vi "HFRR ADV v06.vi"() -> ()   [LabVIEW 2025] (continued)
            n1283 = local read "TEMP"() -> (w1608:dbl)
            n1284 = local write "FF 3"(w1604) -> ()
            n1285 = Compound Arithmetic op=OR("FRICVALZ 4", "FRICVALZ 3", "FRICVALZ 2") -> (w1601:bool)
            n1286 = case shown="True" w1601 {
              tunnel: w1594 -> [_ w1615]
              frame False {
              }
              frame True {
                w1614 = FALSE ("FRICVALZ")
                n1287 = local write "FRICVALZ 3"(w1614) -> ()
                n1288 = local write "FRICVALZ 2"(w1614) -> ()
                n1289 = local write "FRICVALZ 4"(w1614) -> ()
                "FRICVALZ" <- w1615
              }
            }
            n1290 = Not A Number/Path/Refnum?(number/path/refnum=w1608) -> (NaN/Path/Refnum?=w1607:bool)
            n1291 = Not A Number/Path/Refnum?(number/path/refnum=w1604) -> (NaN/Path/Refnum?=w1606:bool)
            n1292 = Divide(x=w1604, y=1.96) -> (x/y=w1591:dbl)
            n1293 = Compound Arithmetic op=OR(w1607, w1606) -> (w1605:bool)
            n1294 = Not A Number/Path/Refnum?(number/path/refnum=w1591) -> (NaN/Path/Refnum?=w1602:bool)
            n1295 = case shown="True" w1605 {
              frame False {
              }
              frame True {
                n1296 = local write "TEMP"(0.0 ("TEMP")) -> ()
                n1297 = local write "FF 2"(0.0 ("FF 2")) -> ()
                n1298 = local write "reinit"(TRUE ("reinit")) -> ()
              }
            }
            n1299 = Select(t=0.0, s=w1602, f=w1591) -> (s? t:f=w1590:dbl)
            "COF 2" <- w1590
            n1300 = local write "COF 3"(w1590) -> ()
          }
        }
      }
    }
    n1301 = Wait (ms)(milliseconds to wait=u32 50) -> ()  [unwired: 1 out]
    n1302 = local read "Quit"() -> (w1530:bool)
    "Rate" <- 2500.0 ("No of Samples")
  }
  n1303 = while {
    tunnel: w57 -> [_]
    tunnel: [w1642] -> _
    tunnel: [w1618] -> w56
    i -> [w1642]
    stop <- w1618 stop-if-true
    # "C:\\LAB-IQ-NXT\\Scar View.exe"
    n1304 = local read "OK Button 16"() -> (w1631:bool)
    n1305 = local read "Main Tab"() -> (w1624:T2)
    n1306 = local read "service 3"() -> (w1625:bool)
    n1307 = local read "OPEN 6"() -> (w1627:bool)
    n1308 = local read "EDIT 2"() -> (w1629:bool)
    n1309 = flat-sequence {
      frame #0 {
        n1310 = local read "SAVE 2"() -> (w2244:bool)
        n1311 = stacked-sequence {
          frame #0 {
            n1312 = local read "EDIT"() -> (w2298:bool)
            n1313 = case shown="True" w2298 {
              tunnel: [u8 2 ("Disabled") u8 0 ("Disabled")] -> _
              frame False {
                w2300 = FALSE
                n1314 = local write "Password"("") -> ()
                n1315 = property on="SrvM CP" class="Bool (strict)"("Visible"=w2300) -> ()  [unwired: 2 in, 2 out]
                n1316 = property on="message" class="Str"("Visible"=w2300) -> ()  [unwired: 2 in, 2 out]
                n1317 = local write "x = y?"(w2300) -> ()
                n1318 = property on="Password" class="Str"("Visible"=w2300) -> ()  [unwired: 2 in, 2 out]
                n1319 = property on="ENTER THE NEW PASSWORD" class="Str"("Visible"=w2300) -> ()  [unwired: 2 in, 2 out]
                n1320 = property on="ENTER CURRENT PASSWORD" class="Str"("Visible"=w2300) -> ()  [unwired: 2 in, 2 out]
                n1321 = local write "SrvM CP"(w2300) -> ()
              }
              frame True {
                w2303 = TRUE
                n1322 = property on="SrvM CP" class="Bool (strict)"("Visible"=w2303) -> ()  [unwired: 2 in, 2 out]
                n1323 = property on="Password" class="Str"("Visible"=w2303) -> ()  [unwired: 2 in, 2 out]
              }
            }
            "dipl pwd" <- "@143$\n" ("dipl pwd")
          }
          frame #1 {
            # "Gain password"
            n1324 = String To Byte Array(string="ENTER CURRENT PASSWORD") -> (unsigned byte array=w2308:u8[])
            n1325 = Search 1D Array(1D array=w2308, element=u8 10) -> (index of element=w2311:i32)  [unwired: 1 in]
            n1326 = Index Array(array=w2308, index=w2311) -> (element=w2307:u8)
            n1327 = Equal?(x=w2307, y=10) -> (x = y?=w2305:bool)
            n1328 = case shown="True" w2305 {
              frame False {
                n1329 = property on="ENTER THE NEW PASSWORD" class="Str"("Visible"=FALSE) -> ()  [unwired: 2 in, 2 out]
              }
              frame True {
                # "password"
                # "change password logic"
                n1330 = local read "ENTER CURRENT PASSWORD"() -> (w2324:string)
                n1331 = local read "dipl pwd"() -> (w2318:string)
                n1332 = String To Byte Array(string=w2324) -> (unsigned byte array=w2326:u8[])
                n1333 = String To Byte Array(string=w2318) -> (unsigned byte array=w2319:u8[])
                n1334 = Array Size(array=w2326) -> (size(s)=w2323:i32)
                n1335 = Array Size(array=w2319) -> (size(s)=w2321:i32)
                n1336 = for {
                  N: w2323 -> [_]
                  tunnel: w2326 -> [w2350]
                  tunnel: [w2348] -> w2327 mode=indexing
                  tunnel: w2323 -> [w2342]
                  i -> [w2343]
                  n1337 = Decrement(x=w2342) -> (x-1=w2340:i32)
                  n1338 = Equal?(x=w2343, y=w2340) -> (x = y?=w2341:bool)
                  n1339 = Index Array(array=w2350, index=w2343) -> (element=w2344:u8)
                  n1340 = Number To Decimal String(number=w2344) -> (decimal integer string=w2349:string)  [unwired: 1 in]
                  n1341 = Select(t="", s=w2341, f="\r") -> (s? t:f=w2346:string)
                  n1342 = Concatenate Strings(w2349, w2346) -> (w2348:string)
                }
                n1343 = for {
                  N: w2321 -> [_]
                  tunnel: w2319 -> [w2338]
                  tunnel: [w2336] -> w2320 mode=indexing
                  tunnel: w2321 -> [w2333]
                  i -> [w2334]
                  n1344 = Decrement(x=w2333) -> (x-1=w2332:i32)
                  n1345 = Equal?(x=w2334, y=w2332) -> (x = y?=w2331:bool)
                  n1346 = Index Array(array=w2338, index=w2334) -> (element=w2337:u8)
                  n1347 = Number To Decimal String(number=w2337) -> (decimal integer string=w2335:string)  [unwired: 1 in]
                  n1348 = Select(t="", s=w2331, f="\r") -> (s? t:f=w2328:string)
                  n1349 = Concatenate Strings(w2335, w2328) -> (w2336:string)
                }
                n1350 = local read "string"() -> (w2325:string)
                n1351 = Concatenate Strings(w2320) -> (w2314:string)
                n1352 = Concatenate Strings(w2325) -> (w2322:string)
                n1353 = Concatenate Strings(w2327) -> (w2315:string)
                n1354 = Equal?(x=w2315, y=w2322) -> (x = y?=w2317:bool)
                n1355 = Equal?(x=w2315, y=w2314) -> (x = y?=w2313:bool)
                n1356 = Or(x=w2317, y=w2313) -> (x .or. y?=w2316:bool)
                n1357 = case shown="True" w2316 {
                  frame False {
                  }
                  frame True {
                    n1358 = property on="ENTER THE NEW PASSWORD" class="Str"("Visible"=TRUE) -> ()  [unwired: 2 in, 2 out]
                  }
                }
              }
            }
          }
          frame #2 {
            n1359 = String To Byte Array(string="ENTER THE NEW PASSWORD") -> (unsigned byte array=w2353:u8[])
            n1360 = Search 1D Array(1D array=w2353, element=u8 10) -> (index of element=w2357:i32)  [unwired: 1 in]
            n1361 = Index Array(array=w2353, index=w2357) -> (element=w2355:u8)
            n1362 = Equal?(x=w2355, y=10) -> (x = y?=w2352:bool)
            n1363 = case shown="False" w2352 {
              frame False {
              }
              frame True {
                n1364 = local write "EDIT"(FALSE) -> ()
                n1365 = local write "SrvM CP"(FALSE) -> ()
                n1366 = local read "ENTER THE NEW PASSWORD"() -> (w2360:string)
                n1367 = String To Byte Array(string=w2360) -> (unsigned byte array=w2365:u8[])
                n1368 = Array Size(array=w2365) -> (size(s)=w2362:i32)
                n1369 = for {
                  N: w2362 -> [_]
                  tunnel: w2365 -> [w2378]
                  tunnel: [w2375] -> w2367 mode=indexing
                  tunnel: w2362 -> [w2370]
                  i -> [w2368]
                  n1370 = Decrement(x=w2370) -> (x-1=w2371:i32)
                  n1371 = Equal?(x=w2368, y=w2371) -> (x = y?=w2372:bool)
                  n1372 = Index Array(array=w2378, index=w2368) -> (element=w2377:u8)
                  n1373 = Number To Decimal String(number=w2377) -> (decimal integer string=w2376:string)  [unwired: 1 in]
                  n1374 = Select(t="", s=w2372, f="\r") -> (s? t:f=w2369:string)
                  n1375 = Concatenate Strings(w2376, w2369) -> (w2375:string)
                }
                n1376 = local read "file path"() -> (w2359:path)
                n1377 = Concatenate Strings(w2367) -> (w2361:string)
                n1378 = Delete(path (use dialog)=w2359) -> (deleted path=w2363:path)  [unwired: 4 in, 2 out]
                n1379 = call <vilib>:"Write Characters To File.vi"("append to file? (new file:F)"=FALSE, "character string"=w2361, "file path (dialog if empty)"=w2363) -> ()  [unwired: 2 in, 1 out]
              }
            }
          }
          frame #3 {
            n1380 = case shown="True" "SrvM CP" {
              frame False {
                w2381 = ""
                n1381 = local write "ENTER CURRENT PASSWORD"(w2381) -> ()
                n1382 = local write "ENTER THE NEW PASSWORD"(w2381) -> ()
                n1383 = property on="ENTER CURRENT PASSWORD" class="Str"("Visible"=FALSE) -> ()  [unwired: 2 in, 2 out]
              }
              frame True {
                n1384 = property on="ENTER THE NEW PASSWORD" class="Str"() -> ("Visible"=w2382:bool)  [unwired: 2 in, 2 out]
                n1385 = Not(x=w2382) -> (.not. x?=w2383:bool)
                n1386 = property on="ENTER CURRENT PASSWORD" class="Str"("Visible"=w2383) -> ()  [unwired: 2 in, 2 out]
              }
            }
          }
          frame #4 {
            n1387 = String To Byte Array(string="Password") -> (unsigned byte array=w2390:u8[])
            n1388 = Search 1D Array(1D array=w2390, element=u8 10) -> (index of element=w2388:i32)  [unwired: 1 in]
            n1389 = Index Array(array=w2390, index=w2388) -> (element=w2389:u8)
            n1390 = Equal?(x=w2389, y=10) -> (x = y?=w2385:bool)
            n1391 = case shown="True" w2385 {
              frame False {
              }
              frame True {
                # "password"
                # "password"
                n1392 = local read "Password"() -> (w2403:string)
                n1393 = String To Byte Array(string=w2403) -> (unsigned byte array=w2406:u8[])
                n1394 = String To Byte Array(string="@143$\n") -> (unsigned byte array=w2392:u8[])
                n1395 = Array Size(array=w2406) -> (size(s)=w2401:i32)
                n1396 = Array Size(array=w2392) -> (size(s)=w2397:i32)
                n1397 = for {
                  N: w2401 -> [_]
                  tunnel: w2406 -> [w2440]
                  tunnel: [w2438] -> w2407 mode=indexing
                  tunnel: w2401 -> [w2435]
                  i -> [w2436]
                  n1398 = Decrement(x=w2435) -> (x-1=w2434:i32)
                  n1399 = Index Array(array=w2440, index=w2436) -> (element=w2439:u8)
                  n1400 = Equal?(x=w2436, y=w2434) -> (x = y?=w2433:bool)
                  n1401 = Number To Decimal String(number=w2439) -> (decimal integer string=w2437:string)  [unwired: 1 in]
                  n1402 = Select(t="", s=w2433, f="\r") -> (s? t:f=w2430:string)
                  n1403 = Concatenate Strings(w2437, w2430) -> (w2438:string)
                }
                n1404 = for {
                  N: w2397 -> [_]
                  tunnel: w2392 -> [w2451]
                  tunnel: [w2449] -> w2395 mode=indexing
                  tunnel: w2397 -> [w2446]
                  i -> [w2447]
                  n1405 = Decrement(x=w2446) -> (x-1=w2445:i32)
                  n1406 = Index Array(array=w2451, index=w2447) -> (element=w2450:u8)
                  n1407 = Equal?(x=w2447, y=w2445) -> (x = y?=w2444:bool)
                  n1408 = Number To Decimal String(number=w2450) -> (decimal integer string=w2448:string)  [unwired: 1 in]
                  n1409 = Select(t="", s=w2444, f="\r") -> (s? t:f=w2441:string)
                  n1410 = Concatenate Strings(w2448, w2441) -> (w2449:string)
                }
                n1411 = local read "file path"() -> (w2391:path)
                n1412 = call <vilib>:"Read Characters From File.vi"("file path (dialog if empty)"=w2391) -> ("character string"=w2405:string)  [unwired: 5 in, 3 out]
                "string" <- w2405
                n1413 = flat-sequence {
                  tunnel: [w2408] -> w2402
                  frame #0 {
                    w2408 = ""
                    n1414 = local write "Password"(w2408) -> ()
                  }
                }
                n1415 = Concatenate Strings(w2395) -> (w2396:string)
                n1416 = Concatenate Strings(w2405) -> (w2404:string)
                n1417 = Concatenate Strings(w2407) -> (w2399:string)
                n1418 = Equal?(x=w2399, y=w2404) -> (x = y?=w2394:bool)
                n1419 = Equal?(x=w2399, y=w2396) -> (x = y?=w2400:bool)
                n1420 = Or(x=w2394, y=w2400) -> (x .or. y?=w2393:bool)
                "x = y?" <- w2393
                n1421 = case shown="True" w2393 {
                  selector: w2393 -> [w2410 _]
                  tunnel: w2402 -> [_ _]
                  frame False {
                    n1422 = And(x=w2410, y=TRUE ("Visible")) -> (x .and. y?=w2411:bool)
                    n1423 = property on="message" class="Str"("Visible"=w2411) -> ()  [unwired: 2 in, 2 out]
                  }
                  frame True {
                    n1424 = control-ref of="This VI"() -> (w2422:refnum<vi>)
                    n1425 = property class="VI"(reference=w2422) -> (reference out=w2413:refnum<vi>, error out=w2417:errorcluster, "Panel"=w2421:refnum<vi>)  [unwired: 1 in]
                    n1426 = property on="message" class="Str"("Visible"=FALSE) -> ()  [unwired: 2 in, 2 out]
                    n1427 = property class="Pnl"(reference=w2421, error in=w2417) -> (reference out=w2415:refnum<vi>, error out=w2418:errorcluster, "Panes[]"=w2420:refnum<vi>[])
                    n1428 = for {
                      tunnel: w2420 -> [w2429] mode=indexing
                      tunnel: T18."Always On" ("Horizontal Scrollbar Visibility") -> [w2428]
                      tunnel: w2418 -> [w2425]
                      tunnel: [w2424] -> w2416
                      n1429 = property class="Pane"(reference=w2429, error in=w2425, "HorizScrollbarVisibility"=w2428) -> (reference out=w2426:refnum<vi>, error out=w2427:errorcluster)
                      n1430 = Close Reference(reference=w2426, error in (no error)=w2427) -> (error out=w2424:errorcluster)
                    }
                    n1431 = Close Reference(reference=w2415, error in (no error)=w2416) -> (error out=w2414:errorcluster)
                    n1432 = Close Reference(reference=w2413, error in (no error)=w2414) -> (error out=→"error out 6":errorcluster)
                  }
                }
              }
            }
          }
        }
        n1433 = local read "x = y?"() -> (w2250:bool)
        n1434 = local read "HUMIDITY: 2"() -> (w2252:dbl)
        n1435 = local read "HUMIDITY:"() -> (w2251:dbl)
        n1436 = property on="Port 2 Error" class="Clust (strict)"("Visible"="EDIT") -> ()  [unwired: 2 in, 2 out]
        n1437 = property on="Port 1 Error" class="Clust (strict)"("Visible"="EDIT") -> ()  [unwired: 2 in, 2 out]
        n1438 = case shown="True" "SrvM CP 2" {
          frame False {
          }
          frame True {
            n1439 = local write "SrvM CP 2"(FALSE ("SrvM CP 2")) -> ()
            n1440 = local read "HUMIDITY: 2"() -> (w2291:dbl)
            n1441 = local read "TEMP INTERCEPT: 2"() -> (w2290:dbl)
            n1442 = local read "DISPLACEMENT : 4"() -> (w2294:dbl)
            n1443 = local read "TEMPERATURE : 2"() -> (w2293:dbl)
            n1444 = local read "STROKE GAIN : 2"() -> (w2295:dbl)
            n1445 = local read "FRIC. FORCE : 2"() -> (w2296:dbl)
            n1446 = local read "AIR TEMP INTERCEPT: 2"() -> (w2289:dbl)
            n1447 = local read "AIR TEMPERATURE : 2"() -> (w2292:dbl)
            n1448 = local write "HUMIDITY:"(w2291) -> ()
            n1449 = local write "AIR TEMP INTERCEPT:"(w2290) -> ()
            n1450 = local write "TEMPERATURE :"(w2293) -> ()
            n1451 = local write "FRIC. FORCE :"(w2296) -> ()
            n1452 = local write "STROKE GAIN :"(w2295) -> ()
            n1453 = local write "DISPLACEMENT :"(w2294) -> ()
            n1454 = local write "AIR TEMPERATURE :"(w2292) -> ()
            n1455 = local write "TEMP INTERCEPT:"(w2289) -> ()
          }
        }
        n1456 = Or(x="SAVE", y=w2244) -> (x .or. y?=w2245:bool)
        n1457 = And(x="EDIT", y=w2250) -> (x .and. y?=w2248:bool)
        n1458 = local read "DISPLACEMENT : 4"() -> (w2261:dbl)
        n1459 = local read "TEMPERATURE : 2"() -> (w2259:dbl)
        n1460 = local read "STROKE GAIN : 2"() -> (w2265:dbl)
        n1461 = local read "DISPLACEMENT :"() -> (w2260:dbl)
        n1462 = local read "FRIC. FORCE : 2"() -> (w2268:dbl)
        n1463 = local read "TEMPERATURE :"() -> (w2257:dbl)
        n1464 = local read "STROKE GAIN :"() -> (w2264:dbl)
        n1465 = local read "FRIC. FORCE :"() -> (w2267:dbl)
        n1466 = case shown="True" w2248 {
          tunnel: [u8 2 ("Disabled") u8 0 ("Disabled")] -> w2247
          tunnel: [w2612 TRUE ("Visible")] -> w2246
          frame False {
            w2612 = FALSE ("Visible")
            n1467 = local write "EDIT 2"(w2612) -> ()
          }
          frame True {
          }
        }
        n1468 = case shown="True" w2245 {
          frame False {
          }
          frame True {
            n1469 = stacked-sequence {
              seq-local: [w2460 _ _] -> [_ w2607 _]
              frame #0 {
                (unwired) i16 5 ("precision (6)")
                # "[CH1]    - FF\n[CH2]   - TEMPERATURE\n[CH3]    - Humidity\n[CH4]    - AIR TEMP\n[CH5]\\- Visa Uno\n[CH6] \\- Visa Due\n[CH7]  \\- file path\n[CH8]   - Displacement Gain\n[CHA]   - Stroke Gain\n[CHB]   - Stroke PID Gain\n[CHC]   -Language Selection\n[CHD]   -Power +\n[CHE]   -Power_\n[CHF]   -Heater\n[CHG]   -Humidity Wet\n[CHH]   -Humidity Dry\n[CHI]   -Integral Time"
                n1470 = local read "Language Selection"() -> (w2508:enum16{"English", "Russian"})
                n1471 = local read "CH-HUMIDITY WET"() -> (w2466:u16)
                n1472 = local read "CH-HUMIDITY DRY"() -> (w2463:u16)
                n1473 = local read "STROKE GAIN :"() -> (w2452:dbl)
                n1474 = local read "CH-POWER +"() -> (w2475:u16)
                n1475 = local read "CH-POWER -"() -> (w2472:u16)
                n1476 = local read "CH-HEATER"() -> (w2469:u16)
                n1477 = local read "AIR TEMPERATURE :"() -> (w2455:dbl)
                n1478 = local read "DISPLACEMENT :"() -> (w2453:dbl)
                n1479 = local read "TEMPERATURE :"() -> (w2456:dbl)
                n1480 = local read "FRIC. FORCE :"() -> (w2457:dbl)
                n1481 = local read "HUMIDITY:"() -> (w2454:dbl)
                n1482 = Path To String(path="File Path") -> (string=w2524:string)
                n1483 = Number To Fractional String(number=w2452, width (-)=i16 10 ("precision (6)"), precision (6)=i16 5) -> (F-format string=w2515:string)  [unwired: 1 in]
                n1484 = Number To Fractional String(number=w2508, width (-)=i16 10 ("precision (6)"), precision (6)=i16 5) -> (F-format string=w2504:string)  [unwired: 1 in]
                n1485 = Number To Fractional String(number=w2475, width (-)=i16 10 ("precision (6)"), precision (6)=i16 5) -> (F-format string=w2498:string)  [unwired: 1 in]
                n1486 = Number To Fractional String(number=w2472, width (-)=i16 10 ("precision (6)"), precision (6)=i16 5) -> (F-format string=w2495:string)  [unwired: 1 in]
                n1487 = Number To Fractional String(number=w2469, width (-)=i16 10 ("precision (6)"), precision (6)=i16 5) -> (F-format string=w2490:string)  [unwired: 1 in]
                n1488 = Number To Fractional String(number=w2466, width (-)=i16 10 ("precision (6)"), precision (6)=i16 5) -> (F-format string=w2487:string)  [unwired: 1 in]
                n1489 = Number To Fractional String(number=w2463, width (-)=i16 10 ("precision (6)"), precision (6)=i16 5) -> (F-format string=w2482:string)  [unwired: 1 in]
                n1490 = local read "Com Port 1"() -> (w2459:refnum<visa-resource-name>)
                n1491 = local read "Com Port 2"() -> (w2458:refnum<visa-resource-name>)
                n1492 = Concatenate Strings(w2524, "\\" ("string")) -> (w2523:string)
                n1493 = Number To Fractional String(number=w2457, width (-)=i16 10 ("precision (6)"), precision (6)=i16 5) -> (F-format string=w2556:string)  [unwired: 1 in]
                n1494 = Number To Fractional String(number=w2456, width (-)=i16 10 ("precision (6)"), precision (6)=i16 5) -> (F-format string=w2555:string)  [unwired: 1 in]
                n1495 = Number To Fractional String(number=w2454, width (-)=i16 10 ("precision (6)"), precision (6)=i16 5) -> (F-format string=w2549:string)  [unwired: 1 in]
                n1496 = Number To Fractional String(number=w2455, width (-)=i16 10 ("precision (6)"), precision (6)=i16 5) -> (F-format string=w2543:string)  [unwired: 1 in]
                n1497 = Number To Fractional String(number=w2453, width (-)=i16 10 ("precision (6)"), precision (6)=i16 5) -> (F-format string=w2516:string)  [unwired: 1 in]
                n1498 = Concatenate Strings("[CHA]" ("string"), w2515, "- Stroke Gain" ("string"), "\r") -> (w2509:string)
                n1499 = Concatenate Strings("[CHC]" ("string"), w2504, "-Language Selection" ("string"), "\r") -> (w2501:string)
                n1500 = Concatenate Strings("[CHD]" ("string"), w2498, "-Power +" ("string"), "\r") -> (w2480:string)
                n1501 = Concatenate Strings("[CHG]" ("string"), w2487, "-Humidity Wet" ("string"), "\r") -> (w2477:string)
                n1502 = Concatenate Strings("[CHH]" ("string"), w2482, "-Humidity Dry" ("string"), "\r") -> (w2476:string)
                n1503 = Concatenate Strings("[CH1]" ("string"), w2556, " - FF" ("string"), "\r") -> (w2554:string)
                n1504 = Concatenate Strings("[CH2]" ("string"), w2555, " - TEMPERATURE" ("string"), "\r") -> (w2553:string)
                n1505 = Concatenate Strings("[CH3]" ("string"), w2549, " - Humidity" ("string"), "\r") -> (w2546:string)
                n1506 = Concatenate Strings("[CH4]" ("string"), w2543, " - AIR TEMP" ("string"), "\r") -> (w2539:string)
                n1507 = Concatenate Strings("[CH5]" ("string"), w2459, "- Visa Uno" ("string"), "\r") -> (w2532:string)
                n1508 = Concatenate Strings("[CH6]" ("string"), w2458, "- Visa Due" ("string"), "\r") -> (w2527:string)
                n1509 = Concatenate Strings("[CH7]" ("string"), w2523, "- file path" ("string"), "\r") -> (w2526:string)
                n1510 = Concatenate Strings("[CH8]" ("string"), w2516, "- Displacement Gain" ("string"), "\r") -> (w2519:string)
                n1511 = Concatenate Strings("[CHE]" ("string"), w2495, "-Power_" ("string"), "\r") -> (w2479:string)
                n1512 = Concatenate Strings("[CHF]" ("string"), w2490, "-Heater" ("string"), "\r") -> (w2478:string)
                n1513 = Concatenate Strings(w2554, w2553, w2546, w2539, w2532, w2527, w2526, w2519, w2509, w2501, w2480, w2479, w2478, w2477, w2476) -> (w2460:string)
                "gain" <- w2460
              }
              frame #1 {
                n1514 = local read "Camera Port :"() -> (w2568:string)
                n1515 = local read "C3 :"() -> (w2576:refnum<visa-resource-name>)
                n1516 = local read "TEMP INTERCEPT:"() -> (w2577:dbl)
                n1517 = local read "AIR TEMP INTERCEPT:"() -> (w2578:dbl)
                n1518 = Concatenate Strings("[CH8]" ("string"), w2568, "- Visa Camera" ("string"), "\r") -> (w2567:string)
                n1519 = Concatenate Strings("[CH7]" ("string"), w2576, "- Visa Humidity" ("string"), "\r") -> (w2572:string)
                n1520 = Number To Fractional String(number=w2577, width (-)=i16 10 ("precision (6)"), precision (6)=i16 5) -> (F-format string=w2595:string)  [unwired: 1 in]
                n1521 = local read "Com Port 3"() -> (w2579:refnum<visa-resource-name>)
                n1522 = Number To Fractional String(number=w2578, width (-)=i16 10 ("precision (6)"), precision (6)=i16 5) -> (F-format string=w2602:string)  [unwired: 1 in]
                n1523 = Concatenate Strings("[CHK]" ("string"), w2595, "-TEMP INTERCEPT" ("string"), "\r") -> (w2591:string)
                n1524 = Concatenate Strings("[SNO]" ("string"), "S.NO", "-" ("string"), "\r") -> (w2587:string)
                n1525 = Concatenate Strings("[CHJ]" ("string"), w2602, "-AIR TEMP INTERCEPT" ("string"), "\r") -> (w2592:string)
                n1526 = Concatenate Strings("[CHL]" ("string"), w2579, "- Visa humid" ("string"), "\r") -> (w2582:string)
                n1527 = String To Path(string="C:\\LAB-IQ\\calibrate WO 2465.dcf") -> (path=w2580:path)
                n1528 = Concatenate Strings(w2607, w2592, w2591, w2587, w2582, w2572, w2567) -> (w2606:string)
                n1529 = call <vilib>:"Write Characters To File.vi"("append to file? (new file:F)"=FALSE, "character string"=w2606, "file path (dialog if empty)"=w2580) -> ()  [unwired: 2 in, 1 out]
              }
              frame #2 {
                n1530 = local write "Lan flag"(0.0 ("Lan flag")) -> ()
                n1531 = local write "conststatus"(0.0 ("rpm value : 2")) -> ()
                n1532 = local write "SAVE"(FALSE ("OK Button 14")) -> ()
                n1533 = local write "SAVE 2"(FALSE ("SAVE 2")) -> ()
              }
            }
          }
        }
        n1534 = Subtract(x=w2252, y=w2251) -> (x-y=w2253:dbl)
        n1535 = local read "AIR TEMPERATURE : 2"() -> (w2256:dbl)
        n1536 = local read "AIR TEMPERATURE :"() -> (w2255:dbl)
        n1537 = Divide(x=w2253, y=w2251) -> (x/y=w2275:dbl)
        n1538 = Subtract(x=w2268, y=w2267) -> (x-y=w2266:dbl)
        n1539 = Subtract(x=w2259, y=w2257) -> (x-y=w2258:dbl)
        n1540 = Subtract(x=w2265, y=w2264) -> (x-y=w2263:dbl)
        n1541 = Subtract(x=w2261, y=w2260) -> (x-y=w2262:dbl)
        n1542 = Subtract(x=w2256, y=w2255) -> (x-y=w2254:dbl)
        n1543 = Divide(x=w2266, y=w2267) -> (x/y=w2286:dbl)
        n1544 = Divide(x=w2258, y=w2257) -> (x/y=w2279:dbl)
        n1545 = Divide(x=w2263, y=w2264) -> (x/y=w2283:dbl)
        n1546 = Divide(x=w2262, y=w2260) -> (x/y=w2282:dbl)
        n1547 = Multiply(x=w2275, y=100.0) -> (x*y=→"HUMIDITY  Calibration Error":dbl)
        n1548 = Divide(x=w2254, y=w2255) -> (x/y=w2278:dbl)
        n1549 = Multiply(x=w2286, y=100.0) -> (x*y=→"FRIC. FORCE Calibration Error":dbl)
        n1550 = Multiply(x=w2279, y=100.0) -> (x*y=→"TEMPERATURE  Calibration Error":dbl)
        n1551 = Multiply(x=w2283, y=100.0) -> (x*y=→"STROKE Calibration Error":dbl)
        n1552 = Multiply(x=w2282, y=100.0) -> (x*y=→"DISPLACEMENT  Calibration Error":dbl)
        n1553 = property on="EDIT 2" class="Bool (strict)"("Visible"=w2246) -> ()  [unwired: 2 in, 2 out]
        n1554 = property on="SAVE" class="Bool (strict)"("Visible"=w2246) -> ()  [unwired: 2 in, 2 out]
        n1555 = property on="SrvM CP" class="Bool (strict)"("Disabled"=w2247) -> ()  [unwired: 2 in, 2 out]
        n1556 = property on="visa due" class="CmbBox"("Disabled"=w2247) -> ()  [unwired: 2 in, 2 out]
        n1557 = property on="File Path" class="Path"("Disabled"=w2247) -> ()  [unwired: 2 in, 2 out]
        n1558 = Multiply(x=w2278, y=100.0) -> (x*y=→"AIR TEMPERATURE  Calibration Error":dbl)
        n1559 = property on="Language Selection" class="Enum (strict)"("Visible"=w2246) -> ()  [unwired: 2 in, 2 out]
        n1560 = property on="Tab Control 7" class="TabCtl (strict)"("Disabled"=w2247) -> ()  [unwired: 2 in, 2 out]
        n1561 = property on="AIR TEMP INTERCEPT:" class="DigNum (strict)"("Disabled"=w2247) -> ()  [unwired: 2 in, 2 out]
        n1562 = property on="CH-POWER -" class="DigNum (strict)"("Disabled"=w2247) -> ()  [unwired: 2 in, 2 out]
        n1563 = property on="CH-POWER +" class="DigNum (strict)"("Disabled"=w2247) -> ()  [unwired: 2 in, 2 out]
        n1564 = property on="AIR TEMPERATURE :" class="DigNum (strict)"("Disabled"=w2247) -> ()  [unwired: 2 in, 2 out]
        n1565 = property on="STROKE GAIN :" class="DigNum (strict)"("Disabled"=w2247) -> ()  [unwired: 2 in, 2 out]
        n1566 = property on="SPEED OUT:" class="DigNum (strict)"("Disabled"=w2247) -> ()  [unwired: 2 in, 2 out]
        n1567 = property on="CH-HUMIDITY DRY" class="DigNum (strict)"("Disabled"=w2247) -> ()  [unwired: 2 in, 2 out]
        n1568 = property on="HUMIDITY:" class="DigNum (strict)"("Disabled"=w2247) -> ()  [unwired: 2 in, 2 out]
        n1569 = property on="CH-HUMIDITY WET" class="DigNum (strict)"("Disabled"=w2247) -> ()  [unwired: 2 in, 2 out]
        n1570 = property on="TEMPERATURE :" class="DigNum (strict)"("Disabled"=w2247) -> ()  [unwired: 2 in, 2 out]
        n1571 = property on="DISPLACEMENT :" class="DigNum (strict)"("Disabled"=w2247) -> ()  [unwired: 2 in, 2 out]
        n1572 = property on="CH-HEATER" class="DigNum (strict)"("Disabled"=w2247) -> ()  [unwired: 2 in, 2 out]
        n1573 = property on="TEMP INTERCEPT:" class="DigNum (strict)"("Disabled"=w2247) -> ()  [unwired: 2 in, 2 out]
        n1574 = property on="FRIC. FORCE :" class="DigNum (strict)"("Disabled"=w2247) -> ()  [unwired: 2 in, 2 out]
      }
    }
    n1575 = local read "RUN"() -> (w1641:bool)
    n1576 = local read "RUN"() -> (w1639:bool)
    n1577 = disable-structure shown="Disabled" {
      disable-tunnel: [w1656 _] -> w1622
      disable-tunnel: [w1655 _] -> w1620
      frame Disabled {
        n1578 = local read "Temperature before test"() -> (w1649:dbl)
        n1579 = local read "Temperature after test"() -> (w1662:dbl)
        n1580 = case shown="True" "Save Results" {
          frame False {
          }
          frame True {
            w1678 = "\r"
            n1581 = local write "Save Results"(FALSE ("OK Button 5")) -> ()
            n1582 = local read "Temperature before test"() -> (w1716:dbl)
            n1583 = local read "Temperature after test"() -> (w1718:dbl)
            n1584 = local read "Humidity before test"() -> (w1715:dbl)
            n1585 = local read "Humidity after test"() -> (w1717:dbl)
            n1586 = local read "WS1.4"() -> (w1722:dbl)
            n1587 = local read "AVP"() -> (w1720:dbl)
            n1588 = Number To Fractional String(number=w1722, width (-)=i16 6, precision (6)=i16 1) -> (F-format string=w1682:string)  [unwired: 1 in]
            n1589 = local read "MWSD"() -> (w1719:dbl)
            n1590 = local read "String"() -> (w1711:string)
            n1591 = local read "FILE"() -> (w1714:string)
            n1592 = local read "HCF"() -> (w1721:dbl)
            n1593 = Number To Fractional String(number=w1715, width (-)=i16 6, precision (6)=i16 1) -> (F-format string=w1707:string)  [unwired: 1 in]
            n1594 = Number To Fractional String(number=w1716, width (-)=i16 6, precision (6)=i16 1) -> (F-format string=w1704:string)  [unwired: 1 in]
            n1595 = Number To Fractional String(number=w1717, width (-)=i16 6, precision (6)=i16 1) -> (F-format string=w1700:string)  [unwired: 1 in]
            n1596 = Number To Fractional String(number=w1718, width (-)=i16 6, precision (6)=i16 1) -> (F-format string=w1696:string)  [unwired: 1 in]
            n1597 = Number To Fractional String(number=w1720, width (-)=i16 6, precision (6)=i16 3) -> (F-format string=w1689:string)  [unwired: 1 in]
            n1598 = Concatenate Strings(w1711, w1714) -> (w1733:string)
            n1599 = Number To Fractional String(number=w1719, width (-)=i16 6, precision (6)=i16 1) -> (F-format string=w1693:string)  [unwired: 1 in]
            n1600 = Number To Fractional String(number=w1721, width (-)=i16 6, precision (6)=i16 2) -> (F-format string=w1687:string)  [unwired: 1 in]
            n1601 = Concatenate Strings("(" ("string"), w1682, ")Microns" ("string")) -> (w1681:string)
            n1602 = local read "REMARKS"() -> (w1713:string)
            "REMARKS 2" <- w1713
            n1603 = Concatenate Strings("(" ("string"), w1707, " ) % RH," ("string")) -> (w1708:string)
            n1604 = Concatenate Strings(w1687, ")" ("string")) -> (w1685:string)
            n1605 = Concatenate Strings("(" ("string"), w1704, ")  Deg C ," ("string")) -> (w1703:string)
            n1606 = Concatenate Strings("(" ("string"), w1700, " ) % RH," ("string")) -> (w1699:string)
            n1607 = Concatenate Strings("(" ("string"), w1696, ")  Deg C ," ("string")) -> (w1695:string)
            n1608 = Concatenate Strings("(" ("string"), w1693, ")  Microns," ("string")) -> (w1692:string)
            n1609 = Concatenate Strings("(" ("string"), w1689, ")  kPa," ("string")) -> (w1679:string)
            n1610 = Concatenate Strings(w1733, ".dwm" ("Substring")) -> (w1731:string)
            n1611 = String To Path(string=w1731) -> (path=w1730:path)
            n1612 = Concatenate Strings(w1713, w1678, " Humidity before test= " ("Substring"), w1708, w1678, " Temperature before test = " ("Substring"), w1703, w1678, " Humidity after test= " ("Substring"), w1699, w1678, "Temperature after test = " ("Substring"), w1695, w1678, "MSD = " ("Substring"), w1692, w1678, "  AVP = " ("Substring"), w1679, w1678, "  HCF                     =( " ("Substring"), w1685, w1678, " WS1.4                  = " ("Substring"), w1681, w1678) -> (w1677:string)
            "data" <- w1677
            n1613 = call <vilib>:"Write Characters To File.vi"("append to file? (new file:F)"=FALSE, "character string"=w1677, "file path (dialog if empty)"=w1730) -> ()  [unwired: 2 in, 1 out]
            n1614 = Match Pattern(string=w1677, regular expression="!") -> (after substring=→"export":string)  [unwired: 1 in, 3 out]
          }
        }
        n1615 = Add(x=231.864, y=w1649) -> (x+y=w1646:dbl)
        n1616 = Add(x=231.864, y=w1662) -> (x+y=w1659:dbl)
        n1617 = Divide(x=1705.984, y=w1646) -> (x/y=w1647:dbl)
        n1618 = Divide(x=1705.984, y=w1659) -> (x/y=w1660:dbl)
        n1619 = local read "Humidity before test"() -> (w1651:dbl)
        n1620 = local read "Humidity after test"() -> (w1664:dbl)
        n1621 = Subtract(x=8.017352 ("y"), y=w1647) -> (x-y=w1673:dbl)
        n1622 = Subtract(x=8.017352 ("y"), y=w1660) -> (x-y=w1667:dbl)
        n1623 = expression code="10**y"(w1673) -> (w1653:dbl)
        n1624 = expression code="10**y"(w1667) -> (w1666:dbl)
        n1625 = Multiply(x=w1651, y=w1653) -> (x*y=w1652:dbl)
        n1626 = Multiply(x=w1664, y=w1666) -> (x*y=w1665:dbl)
        n1627 = Divide(x=w1652, y=750.0) -> (x/y=w1668:dbl)
        n1628 = Divide(x=w1665, y=750.0) -> (x/y=w1669:dbl)
        n1629 = Add(x=w1668, y=w1669) -> (x+y=w1670:dbl)
        n1630 = Divide(x=w1670, y=2.0) -> (x/y=w1672:dbl)
        n1631 = local write "AVP"(w1672) -> ()
        n1632 = Subtract(x=1.4, y=w1672) -> (x-y=w1655:dbl)
        n1633 = local read "HCF"() -> (w1656:dbl)
      }
      frame Enabled {
      }
    }
    n1634 = case shown="True" "EDIT 3" {
      frame False {
      }
      frame True {
        n1635 = local write "EDIT 3"(FALSE ("EDIT 3")) -> ()
        n1636 = local write "Main Tab"(T2."About" ("Main Tab")) -> ()
      }
    }
    n1637 = case shown="False" w1641 {
      frame False {
        n1638 = local read "stopT"() -> (w2619:bool)
        n1639 = case shown="True" w2619 {
          frame False {
          }
          frame True {
            n1640 = local write "stopT"(FALSE) -> ()
          }
        }
      }
      frame True {
        "stopT" <- TRUE
      }
    }
    n1641 = case shown="False" w1639 {
      frame False {
      }
      frame True {
      }
    }
    n1642 = case shown="True" w1629 {
      frame False {
        n1643 = property on="Password 2" class="Str"("Visible"=FALSE) -> ()  [unwired: 2 in, 2 out]
        n1644 = local write "Password 2"("" ("Password")) -> ()
      }
      frame True {
        n1645 = property on="Password 2" class="Str"("Visible"=TRUE) -> ()  [unwired: 2 in, 2 out]
        n1646 = Equal?(x="Password 2", y="HFRR1234") -> (x = y?=w1761:bool)
        n1647 = case shown="True" w1761 {
          tunnel: "Password 2" -> [w1764 _]
          frame False {
            n1648 = String Length(string=w1764) -> (length=w1765:i32)
            n1649 = Greater Than 0?(x=w1765) -> (x > 0?=w1763:bool)
            n1650 = case shown="False" w1763 {
              frame False {
                n1651 = property on="Password 2" class="Str"("Caption.Text"="Password (Advance Setting)") -> ()  [unwired: 2 in, 2 out]
              }
              frame True {
                n1652 = property on="Password 2" class="Str"("Caption.Text"="Incorrect Password!") -> ()  [unwired: 2 in, 2 out]
              }
            }
          }
          frame True {
            (unwired) T26."Advance" ("Main Dashboard Buttons")
            n1653 = local write "EDIT 2"(FALSE ("EDIT 2")) -> ()
            n1654 = local write "Password 2"("" ("Password")) -> ()
            n1655 = local write "Main Tab"(T2."Advance" ("Main Tab")) -> ()
            n1656 = local write "Main Dashboard Buttons"(T1."Advance" ("Main Dashboard Buttons")) -> ()
          }
        }
      }
    }
    n1657 = case shown="True" "Prog Uno" {
      frame False {
      }
      frame True {
        n1658 = stacked-sequence {
          frame #0 {
            n1659 = Delete(path (use dialog)=path "C:/LAB-IQ-NXT/UNOCOMPILE.bat" ("working directory")) -> ()  [unwired: 4 in, 3 out]
          }
          frame #1 {
            n1660 = local read "Com Port 1"() -> (w2226:refnum<visa-resource-name>)
            n1661 = Concatenate Strings("cmd.exe /c \"mode " ("command line"), w2226, ":1200,n,8,1\"\n" ("command line")) -> (w2231:string)
            n1662 = Concatenate Strings(w2231, "CD\\\nCD WinDucom\navrdude -C avrdude.conf -v -patmega328p -carduino -P" ("command line"), w2226, " -b115200 -D -Uflash:w:UNO_V20.hex:i\n" ("command line"), "\r") -> (w2233:string)
            "STR" <- w2233
            n1663 = call <vilib>:"Write Characters To File.vi"("append to file? (new file:F)"=FALSE, "character string"=w2233, "file path (dialog if empty)"=path "C:/LAB-IQ/UNOCOMPILE.bat" ("working directory")) -> ()  [unwired: 2 in, 1 out]
          }
          frame #2 {
            n1664 = disable-structure shown="Disabled" {
              frame Disabled {
                w2237 = "cmd.exe  /c \"C:\\LAB-IQ-NXT\\UNOCOMPILE.bat\"" ("string")
                n1665 = local write "Prog Uno"(FALSE ("run minimized? (F)")) -> ()
                n1666 = call <vilib>:"System Exec.vi"("expected output size  (4096)"=u32 65535, "run minimized? (F)"=FALSE, "wait until completion? (T)"=TRUE ("run minimized? (F)"), "working directory"=path "C:/LAB-IQ-NXT", "standard input"=w2237, "command line"=w2237) -> ("error out"=w2236:errorcluster, "standard output"=→"String 42":string)  [unwired: 2 in, 2 out]
                "error out 3" <- w2236
                n1667 = flat-sequence {
                  tunnel: w2236 -> [_]
                  frame #0 {
                  }
                }
              }
              frame Enabled {
              }
            }
          }
        }
      }
    }
    n1668 = case shown="\"CEC F-096-A-06\"" "TEST STANDARD" {
      tunnel: [2.0 ("Set Temp") 0.0 ("Set Temp") 2.0 ("Set Temp") 0.0 ("Set Temp")] -> w1630
      frame "ASTM D6079", Default {
        w2183 = 50.0 ("Hz")
        w2184 = 53.0 ("Set Rh")
        w2186 = 1.0 ("Set Strk")
        w2185 = 60.0 ("Set Temp")
        # "astm hide"
        n1669 = local write "NORMAL LOAD"(200.0 ("NORMAL LOAD")) -> ()
        n1670 = local write "Set Strk"(w2186) -> ()
        n1671 = local write "Set Hz"(w2183) -> ()
        n1672 = local write "Set Temp"(w2185) -> ()
        n1673 = local write "Set Rh"(w2184) -> ()
        n1674 = local write "test time"(75.0 ("test time")) -> ()
        n1675 = local write "Set Stroke:"(w2186) -> ()
        n1676 = local write "Set Humidity:"(w2184) -> ()
        n1677 = local write "Set Frequency:"(w2183) -> ()
        n1678 = local write "Set Temperature:"(w2185) -> ()
        "Test Standard" <- "ASTM D6079" ("Test Standard 2")
      }
      frame "ISO 12156" {
        n1679 = local write "Set Strk"(1.0 ("Set Strk")) -> ()
        n1680 = local write "NORMAL LOAD"(200.0 ("NORMAL LOAD")) -> ()
        n1681 = local write "Set Temp"(60.0 ("Set Temp")) -> ()
        n1682 = local write "test time"(75.0 ("test time")) -> ()
        n1683 = local write "Set Hz"(50.0 ("Hz")) -> ()
        n1684 = local write "Set Rh"(53.0 ("Set Rh")) -> ()
      }
      frame "CEC F-096-A-06" {
        n1685 = local write "Set Strk"(1.0 ("Set Strk")) -> ()
        n1686 = local write "NORMAL LOAD"(200.0 ("NORMAL LOAD")) -> ()
        n1687 = local write "Set Temp"(60.0 ("Set Temp")) -> ()
        n1688 = local write "test time"(75.0 ("test time")) -> ()
        n1689 = local write "Set Hz"(50.0 ("Hz")) -> ()
        n1690 = local write "Set Rh"(53.0 ("Set Rh")) -> ()
      }
      frame "Custom" {
      }
    }
    n1691 = case shown="True" "Prog Due" {
      frame False {
      }
      frame True {
        n1692 = stacked-sequence {
          frame #0 {
            n1693 = Delete(path (use dialog)=path "C:/LAB-IQ/DUECOMPILE.bat" ("working directory")) -> ()  [unwired: 4 in, 3 out]
          }
          frame #1 {
            n1694 = disable-structure shown="Disabled" {
              frame Disabled {
                n1695 = local read "visa due"() -> (w2208:string)
                n1696 = Concatenate Strings("cmd.exe /c \"mode " ("command line"), w2208, ":1200,n,8,1\"\n" ("command line")) -> (w2213:string)
                n1697 = Concatenate Strings(w2213, "CD\\\nCD WinDucom\nTIMEOUT 1\n bossac.exe -i -d --port=" ("command line"), w2208, " -U false -e -w -v -b DUE.bin -R\n" ("command line"), "\r") -> (w2215:string)
                "concatenated string 2" <- w2215
                n1698 = call <vilib>:"Write Characters To File.vi"("append to file? (new file:F)"=FALSE, "character string"=w2215, "file path (dialog if empty)"=path "C:/LAB-IQ-NXT/DUECOMPILE.bat" ("working directory")) -> ()  [unwired: 2 in, 1 out]
              }
              frame Enabled {
              }
            }
          }
          frame #2 {
            # "C:\\LAB-IQ-NXT\\DUECOMPILE.bat"
            n1699 = disable-structure shown="Disabled" {
              frame Disabled {
                w2220 = "cmd.exe  /c \"C:\\LAB-IQ-NXT\\DUECOMPILE.bat\"" ("string")
                n1700 = call <vilib>:"System Exec.vi"("expected output size  (4096)"=u32 65535, "run minimized? (F)"=FALSE, "wait until completion? (T)"=TRUE ("run minimized? (F)"), "working directory"=path "C:/LAB-IQ-NXT", "standard input"=w2220, "command line"=w2220) -> ("error out"=w2219:errorcluster, "standard output"=→"String 44":string)  [unwired: 2 in, 2 out]
                "error out 4" <- w2219
                n1701 = flat-sequence {
                  tunnel: w2219 -> [_]
                  frame #0 {
                  }
                }
              }
              frame Enabled {
              }
            }
            n1702 = local write "Prog Due"(FALSE ("Prog Due")) -> ()
          }
        }
      }
    }
    n1703 = Or(x=w1627, y=w1625) -> (x .or. y?=w1626:bool)
    n1704 = case shown="\"About\"" w1624 {
      tunnel: [T23."Acquire" ("Main Tab") T23."Compare Files" ("Main Tab") T23."About" ("Main Tab")] -> w1637
      frame "Acquire", Default {
      }
      frame "Compare Files" {
      }
      frame "About" {
      }
    }
    n1705 = Or(x=w1631, y="OPEN") -> (x .or. y?=w1632:bool)
    n1706 = case shown="True" w1632 {
      tunnel: w1631 -> [_ w1772]
      frame False {
      }
      frame True {
        n1707 = stacked-sequence {
          tunnel: w1772 -> [_ w1839 _ _]
          frame #0 {
            w1788 = "  " ("String 6")
            n1708 = local write "OPEN"(FALSE ("open")) -> ()
            n1709 = local read "string1 2"() -> (w1776:string)
            n1710 = local read "string1 3"() -> (w1775:string)
            n1711 = local read "string1 4"() -> (w1774:string)
            n1712 = property on="OPEN" class="Bool (strict)"("Visible"=FALSE) -> ()  [unwired: 2 in, 2 out]
            n1713 = local write "String 6"(w1788) -> ()
            n1714 = local write "String 7"(w1788) -> ()
            n1715 = local write "String 8"(w1788) -> ()
            n1716 = local write "String 12"(w1788) -> ()
            n1717 = local read "OK Button 16"() -> (w1773:bool)
            n1718 = String To Path(string=w1776) -> (path=w1784:path)
            n1719 = String To Path(string=w1775) -> (path=w1783:path)
            n1720 = String To Path(string=w1774) -> (path=w1782:path)
            n1721 = case shown="True" w1773 {
              tunnel: [w1789 w1790] -> w1777
              frame False {
                n1722 = local read "string1"() -> (w1789:string)
              }
              frame True {
                n1723 = local read "String Indicator 4"() -> (w1790:string)
              }
            }
            n1724 = Open/Create/Replace File "Open File"(file path (use dialog)=w1784) -> (refnum out=w1780:refnum<file>)  [unwired: 5 in, 2 out]
            n1725 = Open/Create/Replace File "Open File"(file path (use dialog)=w1783) -> (refnum out=w1779:refnum<file>)  [unwired: 5 in, 2 out]
            n1726 = Open/Create/Replace File "Open File"(file path (use dialog)=w1782) -> (refnum out=w1778:refnum<file>)  [unwired: 5 in, 2 out]
            n1727 = while {
              tunnel: w1780 -> [w1802]
              i -> [w1798]
              stop <- w1797 continue-if-true
              (unwired) TRUE ("line mode (F)")
              n1728 = Read from Text File "Read File"(file (use dialog)=w1802) -> (text=w1799:string)  [unwired: 3 in, 3 out]
              n1729 = local write "Numeric 11"(w1798) -> ()
              n1730 = String Length(string=w1799) -> (length=w1801:i32)
              n1731 = Greater?(x=w1801, y=1) -> (0:w1797:bool)
            }
            n1732 = while {
              tunnel: w1779 -> [w1808]
              i -> [w1804]
              stop <- w1803 continue-if-true
              (unwired) TRUE ("line mode (F)")
              n1733 = Read from Text File "Read File"(file (use dialog)=w1808) -> (text=w1805:string)  [unwired: 3 in, 3 out]
              n1734 = local write "Numeric 12"(w1804) -> ()
              n1735 = String Length(string=w1805) -> (length=w1807:i32)
              n1736 = Greater?(x=w1807, y=1) -> (0:w1803:bool)
            }
            n1737 = while {
              tunnel: w1778 -> [w1814]
              i -> [w1810]
              stop <- w1809 continue-if-true
              (unwired) TRUE ("line mode (F)")
              n1738 = Read from Text File "Read File"(file (use dialog)=w1814) -> (text=w1811:string)  [unwired: 3 in, 3 out]
              n1739 = local write "Numeric 13"(w1810) -> ()
              n1740 = String Length(string=w1811) -> (length=w1813:i32)
              n1741 = Greater?(x=w1813, y=1) -> (0:w1809:bool)
            }
            n1742 = String To Path(string=w1777) -> (path=w1785:path)
            n1743 = Open/Create/Replace File "Open File"(file path (use dialog)=w1785) -> (refnum out=w1781:refnum<file>)  [unwired: 5 in, 2 out]
            n1744 = while {
              tunnel: w1781 -> [w1796]
              i -> [w1792]
              stop <- w1791 continue-if-true
              (unwired) TRUE ("line mode (F)")
              n1745 = Read from Text File "Read File"(file (use dialog)=w1796) -> (text=w1793:string)  [unwired: 3 in, 3 out]
              n1746 = local write "Numeric 8"(w1792) -> ()
              n1747 = String Length(string=w1793) -> (length=w1795:i32)
              n1748 = Greater?(x=w1795, y=1) -> (0:w1791:bool)
            }
          }
          frame #1 {
            w1966 = FALSE ("ACTUAL   MERGE")
            # "Sample Temp"
            # "ECR"
            # "COF"
            # "Time\nCOF\nFF\nTemp"
            n1749 = case shown="True" w1839 {
              tunnel: [w1986 w1987] -> w1840
              frame False {
                n1750 = local read "string1"() -> (w1986:string)
              }
              frame True {
                n1751 = local read "String Indicator 4"() -> (w1987:string)
              }
            }
            n1752 = local read "string1 3"() -> (w1884:string)
            n1753 = String To Path(string=w1840) -> (path=w1971:path)
            n1754 = String To Path(string=w1884) -> (path=w1982:path)
            n1755 = local read "Numeric 12"() -> (w1968:i32)
            n1756 = local read "Numeric 8"() -> (w1970:i32)
            n1757 = local read "string1 2"() -> (w1885:string)
            n1758 = local read "string1 4"() -> (w1883:string)
            n1759 = Open/Create/Replace File "Open File"(file path (use dialog)=w1971) -> (refnum out=w1985:refnum<file>, error out=w1984:errorcluster)  [unwired: 5 in, 1 out]
            n1760 = Open/Create/Replace File "Open File"(file path (use dialog)=w1982) -> (refnum out=w1978:refnum<file>, error out=w1979:errorcluster)  [unwired: 5 in, 1 out]
            n1761 = for {
              N: w1970 -> [_]
              tunnel: w1985 -> [w2133]
              tunnel: w1984 -> [w2132]
              tunnel: [w2122] -> w1897 mode=indexing
              tunnel: [w2120] -> w1954 mode=indexing
              tunnel: [w2121] -> w1949 mode=indexing
              tunnel: w1966 -> [_]
              tunnel: [w2114] -> w1951 mode=indexing
              tunnel: [w2110] -> w1920 mode=indexing
              tunnel: [w2106] -> w1895 mode=indexing
              tunnel: [w2102] -> w1876 mode=indexing
              tunnel: [w2097] -> w1836 mode=indexing
              (unwired) TRUE ("line mode (F)")
              # "freq"
              # "Stroke"
              # "Time"
              # "CoF"
              # "Humidity"
              # "Temp"
              # "Air Temp"
              # "ECR"
              n1762 = Read from Text File "Read File"(file (use dialog)=w2133, error in=w2132) -> (text=w2098:string)  [unwired: 2 in, 3 out]
              n1763 = local write "String 6"(w2098) -> ()
              n1764 = String Subset(string=w2098, offset (0)=0, length (rest)=14 ("length (rest)")) -> (substring=w2126:string)
              n1765 = String Subset(string=w2098, offset (0)=35, length (rest)=9 ("length (rest)")) -> (substring=w2123:string)
              n1766 = String Subset(string=w2098, offset (0)=15, length (rest)=9 ("length (rest)")) -> (substring=w2129:string)
              n1767 = Fract/Exp String To Number(string=w2126) -> (number=w2122:dbl)  [unwired: 3 in, 1 out]
              n1768 = Fract/Exp String To Number(string=w2123) -> (number=w2121:dbl)  [unwired: 3 in, 1 out]
              n1769 = Fract/Exp String To Number(string=w2129) -> (number=w2120:dbl)  [unwired: 3 in, 1 out]
              n1770 = String Subset(string=w2098, offset (0)=85, length (rest)=9 ("length (rest)")) -> (substring=w2099:string)
              n1771 = String Subset(string=w2098, offset (0)=25, length (rest)=9 ("length (rest)")) -> (substring=w2105:string)
              n1772 = String Subset(string=w2098, offset (0)=55, length (rest)=9 ("length (rest)")) -> (substring=w2107:string)
              n1773 = String Subset(string=w2098, offset (0)=45, length (rest)=9 ("length (rest)")) -> (substring=w2113:string)
              n1774 = String Subset(string=w2098, offset (0)=65, length (rest)=9 ("length (rest)")) -> (substring=w2119:string)
              n1775 = Fract/Exp String To Number(string=w2105) -> (number=w2102:dbl)  [unwired: 3 in, 1 out]
              n1776 = Fract/Exp String To Number(string=w2099) -> (number=w2097:dbl)  [unwired: 3 in, 1 out]
              n1777 = Fract/Exp String To Number(string=w2107) -> (number=w2106:dbl)  [unwired: 3 in, 1 out]
              n1778 = Fract/Exp String To Number(string=w2113) -> (number=w2110:dbl)  [unwired: 3 in, 1 out]
              n1779 = Fract/Exp String To Number(string=w2119) -> (number=w2116:dbl)  [unwired: 3 in, 1 out]
              n1780 = Add(x=w2116, y=0.0) -> (x+y=w2114:dbl)
            }
            n1781 = for {
              N: w1968 -> [_]
              tunnel: w1979 -> [w2059]
              tunnel: w1978 -> [w2058]
              tunnel: [w2048] -> w1937 mode=indexing
              tunnel: [w2046] -> w1935 mode=indexing
              tunnel: [w2047] -> w1931 mode=indexing
              tunnel: w1966 -> [_]
              tunnel: [w2040] -> w1933 mode=indexing
              tunnel: [w2036] -> w1915 mode=indexing
              tunnel: [w2032] -> w1891 mode=indexing
              tunnel: [w2029] -> w1872 mode=indexing
              tunnel: [w2025] -> w1831 mode=indexing
              (unwired) 9 ("length (rest)")
              (unwired) 9 ("length (rest)")
              (unwired) TRUE ("line mode (F)")
              n1782 = Read from Text File "Read File"(file (use dialog)=w2058, error in=w2059) -> (text=w2026:string)  [unwired: 2 in, 3 out]
              n1783 = local write "String 8"(w2026) -> ()
              n1784 = String Subset(string=w2026, offset (0)=85) -> (substring=w2028:string)  [unwired: 1 in]
              n1785 = String Subset(string=w2026, offset (0)=35, length (rest)=9 ("length (rest)")) -> (substring=w2049:string)
              n1786 = String Subset(string=w2026, offset (0)=55, length (rest)=9 ("length (rest)")) -> (substring=w2034:string)
              n1787 = String Subset(string=w2026, offset (0)=25) -> (substring=w2030:string)  [unwired: 1 in]
              n1788 = String Subset(string=w2026, offset (0)=15, length (rest)=9 ("length (rest)")) -> (substring=w2055:string)
              n1789 = String Subset(string=w2026, offset (0)=0, length (rest)=14 ("length (rest)")) -> (substring=w2052:string)
              n1790 = String Subset(string=w2026, offset (0)=45, length (rest)=9 ("length (rest)")) -> (substring=w2039:string)
              n1791 = String Subset(string=w2026, offset (0)=65, length (rest)=9 ("length (rest)")) -> (substring=w2045:string)
              n1792 = Fract/Exp String To Number(string=w2028) -> (number=w2025:dbl)  [unwired: 3 in, 1 out]
              n1793 = Fract/Exp String To Number(string=w2049) -> (number=w2047:dbl)  [unwired: 3 in, 1 out]
              n1794 = Fract/Exp String To Number(string=w2034) -> (number=w2032:dbl)  [unwired: 3 in, 1 out]
              n1795 = Fract/Exp String To Number(string=w2030) -> (number=w2029:dbl)  [unwired: 3 in, 1 out]
              n1796 = Fract/Exp String To Number(string=w2055) -> (number=w2046:dbl)  [unwired: 3 in, 1 out]
              n1797 = Fract/Exp String To Number(string=w2052) -> (number=w2048:dbl)  [unwired: 3 in, 1 out]
              n1798 = Fract/Exp String To Number(string=w2039) -> (number=w2036:dbl)  [unwired: 3 in, 1 out]
              n1799 = Fract/Exp String To Number(string=w2045) -> (number=w2042:dbl)  [unwired: 3 in, 1 out]
              n1800 = Add(x=w2042, y=0.0) -> (x+y=w2040:dbl)
            }
            n1801 = String To Path(string=w1885) -> (path=w1983:path)
            n1802 = String To Path(string=w1883) -> (path=w1977:path)
            n1803 = local read "Numeric 11"() -> (w1967:i32)
            n1804 = local read "Numeric 13"() -> (w1969:i32)
            n1805 = Open/Create/Replace File "Open File"(file path (use dialog)=w1983) -> (refnum out=w1981:refnum<file>, error out=w1980:errorcluster)  [unwired: 5 in, 1 out]
            n1806 = Open/Create/Replace File "Open File"(file path (use dialog)=w1977) -> (refnum out=w1976:refnum<file>, error out=w1975:errorcluster)  [unwired: 5 in, 1 out]
